vi "Write to File Last Update Information ver2.vi"(7 "Shift":string, 8 "error in":errorcluster, 11 "Refnum in":T1) -> (0 "error out":errorcluster, 3 "refnum out":T1)   [LabVIEW 2018]
uses:
  <vilib>/Utility/config.llb/Config Data RefNum.ctl
  <vilib>/Utility/config.llb/Write Key (String).vi
  <vilib>/Utility/config.llb/NI_LVConfig.lvlib
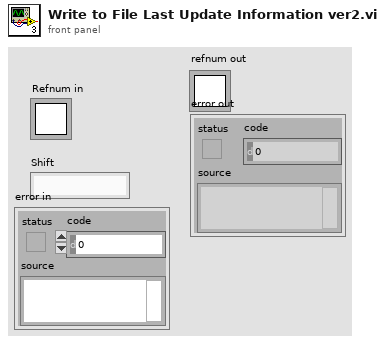
[diagram p1: front panel]
types:
  T1 = typedef "NI_LVConfig.lvlib/Config Data RefNum.ctl" = refnum<k1>
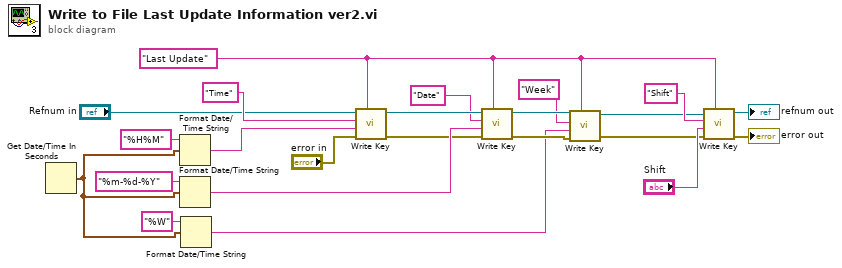
[diagram p0: block diagram]
diagram:
  w5 = "Last Update" ("section")
  n1 = Get Date/Time In Seconds() -> (seconds since 1Jan1904=w3:timestamp)
  n2 = Format Date/Time String(time format string (%c)="%H%M", seconds (now)=w3) -> (date/time string=w16:string)  [unwired: 1 in]
  n3 = Format Date/Time String(time format string (%c)="%m-%d-%Y", seconds (now)=w3) -> (date/time string=w21:string)  [unwired: 1 in]
  n4 = Format Date/Time String(time format string (%c)="%W", seconds (now)=w3) -> (date/time string=w2:string)  [unwired: 1 in]
  n5 = call-poly <vilib>:"Write Key.vi"("section"=w5, "error in (no error)"="error in", "value"=w16, "key"="Time", "refnum"="Refnum in") -> ("error out"=w20:errorcluster, "refnum out"=w19:T1)  [unwired: 4 in, 1 out]
  n6 = call-poly <vilib>:"Write Key.vi"("section"=w5, "error in (no error)"=w20, "value"=w21, "key"="Date", "refnum"=w19) -> ("error out"=w8:errorcluster, "refnum out"=w9:T1)  [unwired: 4 in, 1 out]
  n7 = call-poly <vilib>:"Write Key.vi"("section"=w5, "error in (no error)"=w8, "value"=w2, "key"="Week", "refnum"=w9) -> ("error out"=w6:errorcluster, "refnum out"=w7:T1)  [unwired: 4 in, 1 out]
  n8 = call-poly <vilib>:"Write Key.vi"("section"=w5, "error in (no error)"=w6, "value"="Shift", "key"="Shift", "refnum"=w7) -> ("error out"=→"error out":errorcluster, "refnum out"=→"refnum out":T1)  [unwired: 4 in, 1 out]
